vi "CANXNETRead.vi"(11 "XNET":T1) -> (0 "Frame":cluster{"ID":u32, "Data":u8[]}[](array[cluster]), 3 "XNET out":T1)   [LabVIEW 2017]
doc: "This example demonstrates frame streaming input using an NI-XNET Frame Input session. \n\nThis example can run against any output example, assuming you have a properly terminated CAN cable connected to two CAN ports.\n\nIf you have no database aliases on your system, the example automatically loads the nixnet_example database."
uses:
  <vilib>/xnet/xnet.llb/XNET Read (Frame CAN).vi
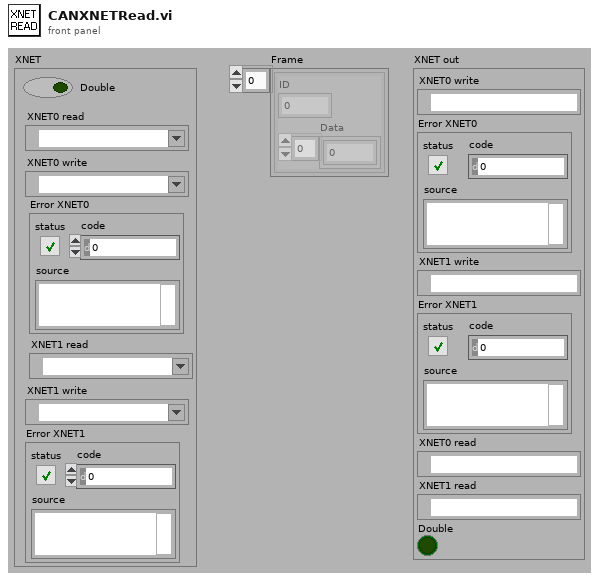
[diagram p1: front panel]
types:
  T1 = cluster{"XNET0 write":refnum<k21>, "Error XNET0":errorcluster, "XNET1 write":refnum<k21>, "Error XNET1":errorcluster, "XNET0 read":refnum<k21>, "XNET1 read":refnum<k21>, "Double":bool}
  T2 = typedef "XNET Frame CAN.ctl" = cluster{"timestamp":timestamp, "payload":u8[], "identifier":u32, "type":T3, "extended?":bool, "echo?":bool}
  T3 = typedef "XNET Frame Type CAN.ctl" = u8
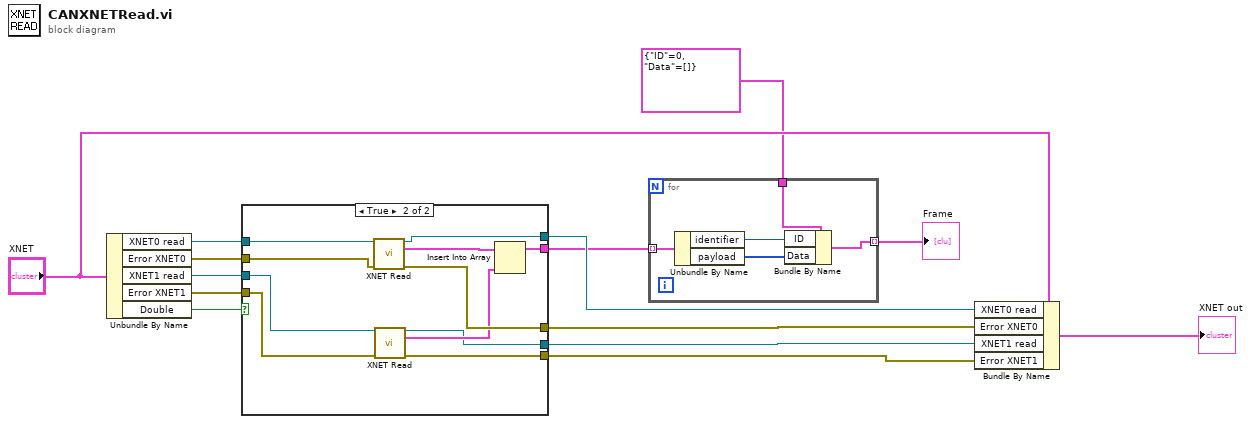
[diagram p0: block diagram]
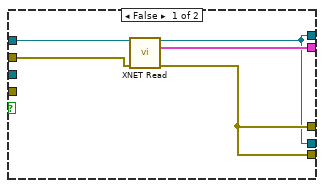
[diagram p2: hidden frame]
diagram:
  n1 = Unbundle By Name("XNET") -> ("XNET0 read"=w14:refnum<k21>, "Error XNET0"=w13:errorcluster, "XNET1 read"=w12:refnum<k21>, "Error XNET1"=w11:errorcluster, "Double"=w8:bool)
  n2 = case shown="True" w8 {
    tunnel: [w18 w23] -> w3
    tunnel: w14 -> [w19 w30]
    tunnel: w13 -> [w15 w29]
    tunnel: w12 -> [_ w28]
    tunnel: w11 -> [_ w27]
    tunnel: [w17 w26] -> w9
    tunnel: [w17 w25] -> w6
    tunnel: [w16 w21] -> w5
    tunnel: [w16 w20] -> w4
    frame False {
      n3 = call-poly <vilib>:"XNET Read.vi"("session in"=w19, "error in (no error)"=w15) -> ("session out"=w16:refnum<k21>, "data"=w18:T2[], "error out"=w17:errorcluster)  [unwired: 11 out]
    }
    frame True {
      n4 = call-poly <vilib>:"XNET Read.vi"("session in"=w30, "error in (no error)"=w29) -> ("session out"=w21:refnum<k21>, "data"=w24:T2[], "error out"=w26:errorcluster)  [unwired: 11 out]
      n5 = call-poly <vilib>:"XNET Read.vi"("session in"=w28, "error in (no error)"=w27) -> ("session out"=w20:refnum<k21>, "data"=w22:T2[], "error out"=w25:errorcluster)  [unwired: 11 out]
      n6 = Insert Into Array(array=w24, new element=w22) -> (w23:T2[])  [unwired: 1 in]
    }
  }
  n7 = for {
    tunnel: w3 -> [w35] mode=indexing
    tunnel: cluster{"ID":u32, "Data":u8[]} {"ID"=0, "Data"=[]} -> [w34]
    tunnel: [w31] -> w1 mode=indexing
    n8 = Unbundle By Name(w35) -> ("identifier"=w33:u32, "payload"=w32:u8[])
    n9 = Bundle By Name(cluster=w34, "ID"=w33, "Data"=w32) -> (w31:cluster{"ID":u32, "Data":u8[]})
  }
  "Frame" <- w1
  n10 = Bundle By Name(cluster="XNET", "XNET0 read"=w5, "Error XNET0"=w9, "XNET1 read"=w4, "Error XNET1"=w6) -> (→"XNET out":T1)
